vi "Delete From Array.vi"() -> ()   [LabVIEW 2017]
panel:
  out "Split Array":dbl[](array[numeric])
  in  "Length":i32
  in  "index":i32
  in  "Boolean":bool
  out "deleted portion":dbl
  out "array w/ subset deleted":dbl[](array[numeric])
  in  "array":dbl[](array[numeric])
  # "Delete From Array"
  # "If Boolean is true, deletes the Number  from the Array based on the Index input. If the Boolean is false, splits the array starting at Element Index, creating two separate arrays."
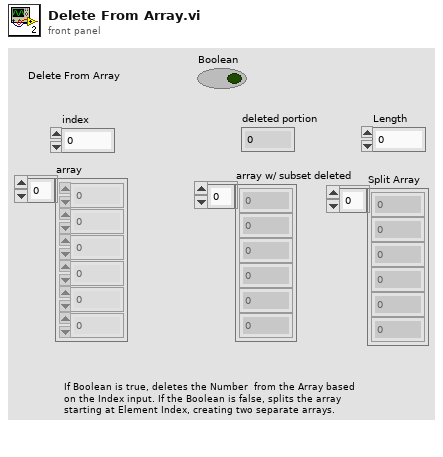
[diagram p1: front panel]
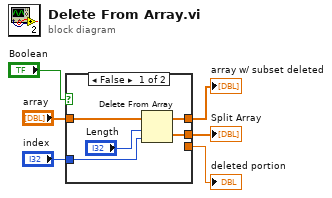
[diagram p0: block diagram]
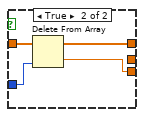
[diagram p2: hidden frame]
diagram:
  n1 = case shown="False" "Boolean" {
    tunnel: "array" -> [w11 w15]
    tunnel: [w10 w14] -> w5
    tunnel: [_ w13] -> w4
    tunnel: "index" -> [w9 w12]
    tunnel: [w7 _] -> w1
    frame False {
      n2 = Delete From Array(array=w11, length="Length", index=w9) -> (deleted portion=w7:dbl[], array with subset deleted=w10:dbl[])
    }
    frame True {
      n3 = Delete From Array(array=w15, index=w12) -> (deleted portion=w13:dbl, array with subset deleted=w14:dbl[])  [unwired: 1 in]
    }
  }
  "array w/ subset deleted" <- w5
  "deleted portion" <- w4
  "Split Array" <- w1
